vi "Sampling Stats.vi"(11 "Waveform in":waveform(dbl)) -> (0 "Samples per iteration":dbl, 1 "Sampling period":dbl, 2 "Sampling frequency":dbl, 3 "Number of samples":dbl format="%0.2f")   [LabVIEW 2014, in "Aquisicao de Dados.lvlib"]
uses:
  Aquisicao de Dados.lvlib
  <vilib>/Waveform/WDTOps.llb/WDT Number of Waveform Samples DBL.vi
  <vilib>/Waveform/WDTOps.llb/WDT Waveform Duration DBL.vi
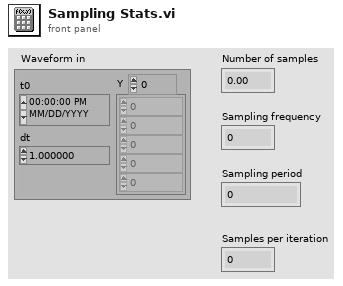
[diagram p1: front panel]
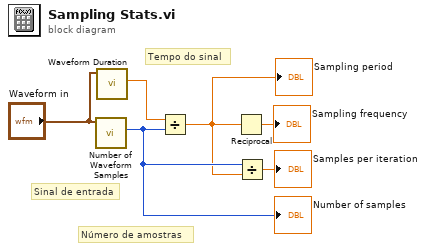
[diagram p0: block diagram]
diagram:
  # "Sinal de entrada"
  # "Número de amostras"
  # "Tempo do sinal"
  n1 = call-poly <vilib>:"Number of Waveform Samples.vi"("waveform in"="Waveform in") -> ("number of samples"=w2:i32)  [unwired: 8 in, 2 out]
  "Number of samples" <- w2
  n2 = call-poly <vilib>:"Waveform Duration.vi"("waveform in"="Waveform in") -> ("duration"=w5:dbl)  [unwired: 8 in, 2 out]
  n3 = Divide(x=w5, y=w2) -> (x/y=w1:dbl)
  "Sampling period" <- w1
  n4 = Reciprocal(x=w1) -> (1/x=→"Sampling frequency":dbl)
  n5 = Divide(x=w2, y=w1) -> (x/y=→"Samples per iteration":dbl)
